vi "search_lc_tb.vi"(8 "neirong":string, 11 "id":string) -> (0 "error":errorcluster caption="error out 4", 1 "data":string[][](array[string]) caption="查询数据")   [LabVIEW 2017, in "Lib_code.lvlib"]
uses:
  Lib_code.lvlib
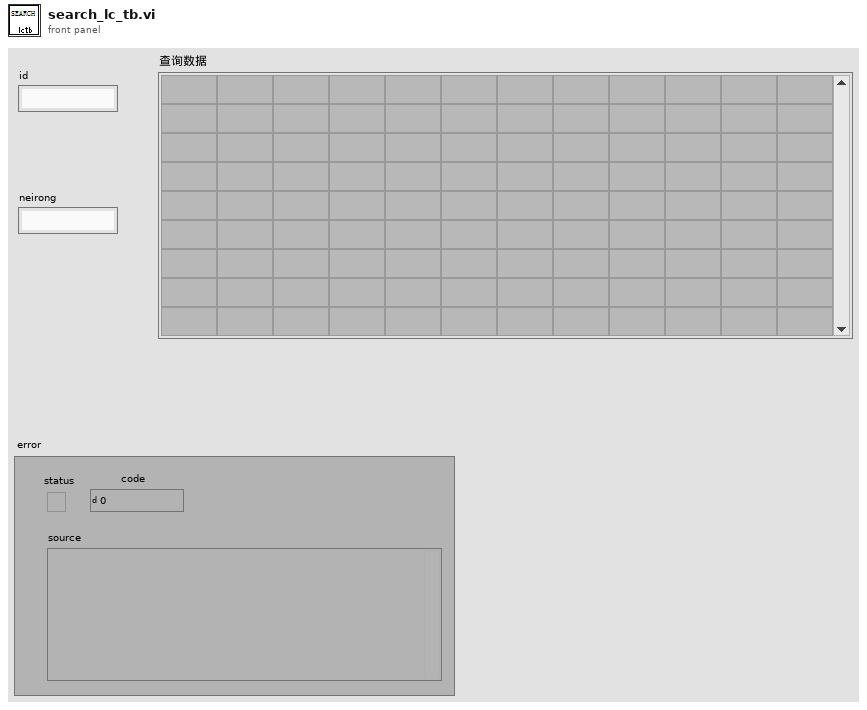
[diagram p1: front panel]
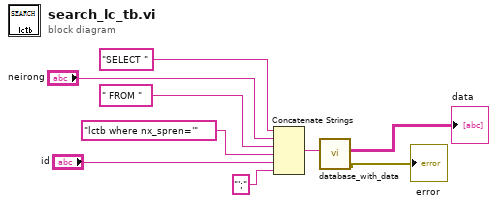
[diagram p0: block diagram]
diagram:
  n1 = Concatenate Strings("SELECT " ("格式字符串"), "neirong", " FROM " ("格式字符串"), "lctb where nx_spren='" ("格式字符串"), "id", "';" ("字符串")) -> (w3:string)
  n2 = call "database_with_data.vi"("input"=w3) -> ("error"=→"error":errorcluster, "Data"=→"data":string[][])  [unwired: 9 in]
